vi "5_1.vi"() -> ()   [LabVIEW 2018]
uses:
  <vilib>/ptbypt/NI_PtbyPt.lvlib
  <vilib>/gmath/NI_Gmath.lvlib
panel:
  out "统计门限判决正确数":u64
  out "理论门限正确数":u64
  out "理论误码率":dbl
  out "噪声标准差":dbl
  out "理论门限误码率":dbl
  out "统计门限误码率":dbl
  out "理论最优门限":dbl
  out "统计最优门限":dbl
  out "先验概率P(H1)":dbl
  in  "先验概率P(H0)":dbl=0.46
  in  "噪声方差":dbl=0.02
  in  "样本数":u64=1000000
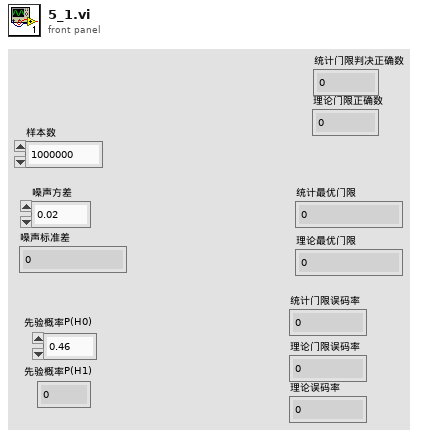
[diagram p1: front panel]
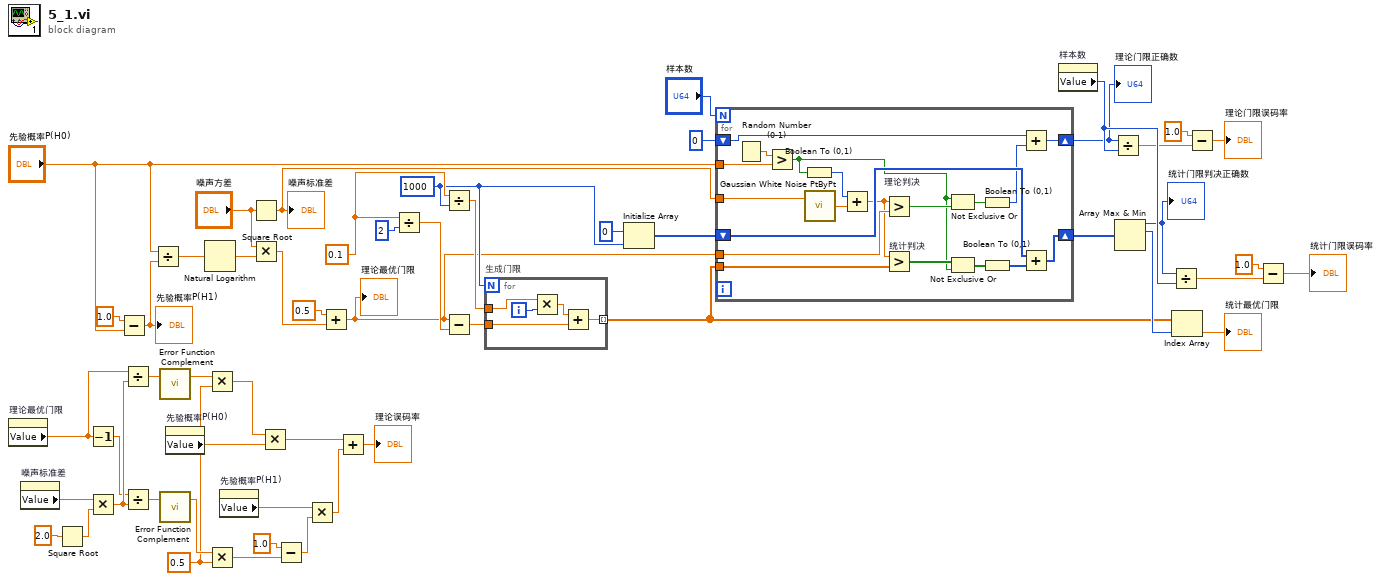
[diagram p0: block diagram]
diagram:
  w16 = 0.5 ("y")
  w42 = 0.1 ("x")
  w34 = u64 1000
  n1 = property on="理论最优门限" class="DigNum (严格)"() -> ("Value"=w22:dbl)  [unwired: 2 in, 2 out]
  n2 = property on="噪声标准差" class="DigNum (严格)"() -> ("Value"=w25:dbl)  [unwired: 2 in, 2 out]
  n3 = Square Root(x=2.0) -> (sqrt(x)=w24:dbl)
  n4 = Decrement(x=w22) -> (x-1=w21:dbl)
  n5 = Multiply(x=w25, y=w24) -> (x*y=w23:dbl)
  n6 = Subtract(x=1.0, y="先验概率P(H0)") -> (x-y=w33:dbl)
  "先验概率P(H1)" <- w33
  n7 = Divide(x=w22, y=w23) -> (x/y=w20:dbl)
  n8 = Divide(x=w21, y=w23) -> (x/y=w19:dbl)
  n9 = Divide(x="先验概率P(H0)", y=w33) -> (x/y=w51:dbl)
  n10 = call <vilib>:"Error Function Complement.vi"("x"=w20) -> ("1 - erf(x)"=w17:dbl)  [unwired: 2 in]
  n11 = call <vilib>:"Error Function Complement.vi"("x"=w19) -> ("1 - erf(x)"=w18:dbl)  [unwired: 2 in]
  n12 = property on="先验概率P(H0)" class="DigNum (严格)"() -> ("Value"=w5:dbl)  [unwired: 2 in, 2 out]
  n13 = Natural Logarithm(1:w51) -> (0:w50:dbl)
  n14 = Multiply(x=w17, y=w16) -> (x*y=w6:dbl)
  n15 = Multiply(x=w18, y=w16) -> (x*y=w15:dbl)
  n16 = property on="先验概率P(H1)" class="DigNum (严格)"() -> ("Value"=w4:dbl)  [unwired: 2 in, 2 out]
  n17 = Square Root(x="噪声方差") -> (sqrt(x)=w27:dbl)
  "噪声标准差" <- w27
  n18 = Multiply(x="噪声方差", y=w50) -> (x*y=w49:dbl)
  n19 = Multiply(x=w6, y=w5) -> (x*y=w1:dbl)
  n20 = Subtract(x=1.0, y=w15) -> (x-y=w3:dbl)
  n21 = Multiply(x=w4, y=w3) -> (x*y=w2:dbl)
  n22 = Add(x=0.5, y=w49) -> (x+y=w30:dbl)
  "理论最优门限" <- w30
  n23 = Add(x=w1, y=w2) -> (x+y=→"理论误码率":dbl)
  n24 = Divide(x=w42, y=u64 2) -> (x/y=w43:dbl)
  n25 = Divide(x=w42, y=w34) -> (x/y=w45:dbl)
  n26 = Subtract(x=w30, y=w43) -> (x-y=w44:dbl)
  n27 = for "生成门限" {
    N: w34 -> [_]
    tunnel: w45 -> [w57]
    tunnel: [w55] -> w35 mode=indexing
    tunnel: w44 -> [w54]
    i -> [w58]
    n28 = Multiply(x=w57, y=w58) -> (x*y=w56:dbl)
    n29 = Add(x=w56, y=w54) -> (x+y=w55:dbl)
  }
  n30 = Initialize Array(u64 0 ("元素"), w34) -> (w39:u64[])
  n31 = for {
    N: "样本数" -> [_]
    tunnel: w27 -> [w77]
    tunnel: "先验概率P(H0)" -> [w74]
    tunnel: w35 -> [w73]
    shift-right: [w70] -> w37
    shift-left: w39 -> [w71]
    tunnel: w30 -> [w68]
    shift-right: [w66] -> w28
    shift-left: u64 0 ("元素") -> [w64]
    n32 = Random Number (0-1)() -> (number: 0 to 1=w75:dbl)
    n33 = Greater?(x=w75, y=w74) -> (0:w59:bool)
    n34 = Boolean To (0,1)(Boolean=w59) -> (0, 1=w63:i16)
    n35 = call <vilib>:"Gaussian White Noise PtByPt.vi"("standard deviation"=w77) -> ("Gaussian white noise"=w76:dbl)  [unwired: 2 in]
    n36 = Add(x=w63, y=w76) -> (x+y=w60:dbl)
    n37 = Greater? "理论判决"(x=w60, y=w68) -> (0:w67:bool)
    n38 = Greater? "统计判决"(x=w60, y=w73) -> (0:w69:bool[])
    n39 = Not Exclusive Or(1:w67, 2:w59) -> (0:w62:bool)
    n40 = Not Exclusive Or(1:w59, 2:w69) -> (0:w61:bool[])
    n41 = Boolean To (0,1)(Boolean=w62) -> (0, 1=w65:i16)
    n42 = Boolean To (0,1)(Boolean=w61) -> (0, 1=w72:i16[])
    n43 = Add(x=w64, y=w65) -> (x+y=w66:u64)
    n44 = Add(x=w71, y=w72) -> (x+y=w70:u64[])
  }
  "理论门限正确数" <- w28
  n45 = property on="样本数" class="DigNum (严格)"() -> ("Value"=w31:u64)  [unwired: 2 in, 2 out]
  n46 = Divide(x=w28, y=w31) -> (x/y=w9:dbl)
  n47 = Array Max & Min(array=w37) -> (max value=w29:u64, max index (indices)=w36:i32)  [unwired: 2 out]
  "统计门限判决正确数" <- w29
  n48 = Divide(x=w29, y=w31) -> (x/y=w12:dbl)
  n49 = Index Array(array=w35, index=w36) -> (element=→"统计最优门限":dbl)
  n50 = Subtract(x=1.0, y=w9) -> (x-y=→"理论门限误码率":dbl)
  n51 = Subtract(x=1.0, y=w12) -> (x-y=→"统计门限误码率":dbl)
